vi "bullet type msg.vi"(10 "bullet type":i32) -> (2 "String":string)   [LabVIEW 2025]
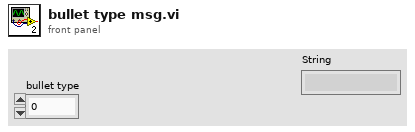
[diagram p1: front panel]
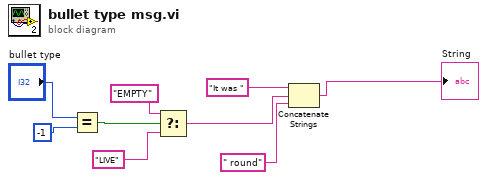
[diagram p0: block diagram]
diagram:
  n1 = Equal?(x="bullet type", y=-1) -> (x = y?=w7:bool)
  n2 = Select(t="EMPTY", s=w7, f="LIVE") -> (s? t:f=w4:string)
  n3 = Concatenate Strings("It was ", w4, " round") -> (→"String":string)
